vi "Log VNA Data - mat.vi"(4 "error in (no error)":errorcluster, 7 "Data in":T1 {"LogStartTime" format="%<%x %.3X>T"}) -> (0 "error out":errorcluster, 3 "Data out":T1 {"LogStartTime" format="%<%x %.3X>T"})   [LabVIEW 2023]
uses:
  controls/UI Data.ctl
  <vilib>/NI/Modbus Library/API/Master/Modbus Master.lvclass
  LibreVNA/LibreVNA.lvclass
  <vilib>/Platform/storage/Storage.llb/usiSequenceRepresentation.ctl
  <vilib>/Platform/storage/lvStorage.llb/_createOrGetByNameExplicitChildObject.vi
  <vilib>/Platform/storage/Storage.llb/__savePropString.vi
  <vilib>/Platform/storage/lvStorage.llb/xStorage/xStorageSupp/ErrorOut.vi
  <vilib>/Platform/storage/lvStorage.llb/_saveFloat64Channel.vi
  <vilib>/Platform/storage/lvStorage.llb/xStorage/Write Data/Write Data.xnode
panel:
  out "resulting string":string
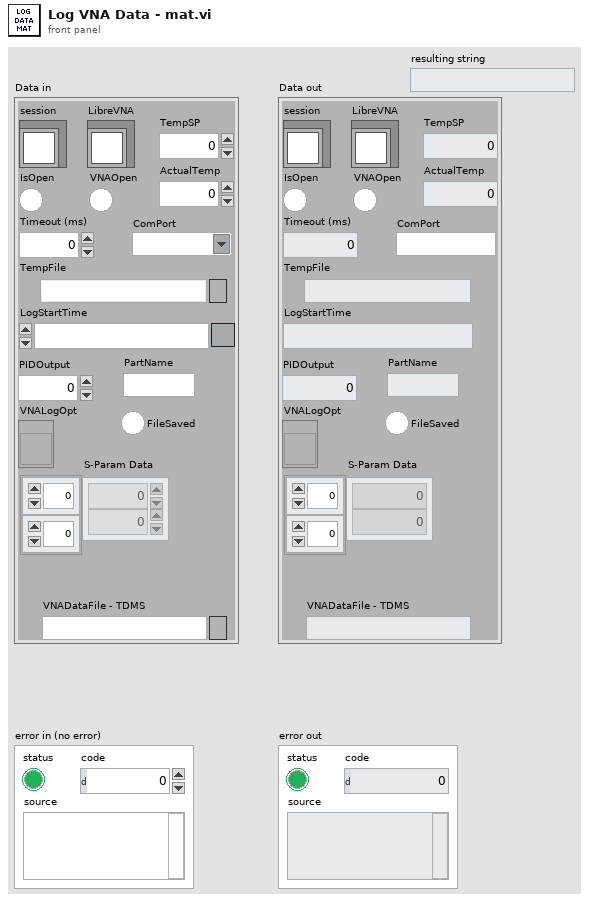
[diagram p1: front panel]
types:
  T1 = typedef "UI Data.ctl" = cluster{"session":refnum<class "Modbus Master.lvclass">, "IsOpen":bool, "Timeout (ms)":i32, "TempFile":path, "LogStartTime":timestamp, "LibreVNA":refnum<class "LibreVNA.lvclass">, "VNAOpen":bool, "TempSP":dbl, "ActualTemp":dbl, "FileSaved":bool, "PIDOutput":dbl, "VNALogOpt":refnum<vi>, "PartName":string, "ComPort":refnum<visa-resource-name>, "S-Param Data":dbl[][], "VNADataFile - TDMS":path}
  T2 = enum16{"Append values", "Replace values at index", "Replace all values"}
  T3 = enum16{"UPDATE", "READ", "QUERY", "CREATE CHILD", "CREATE", "CONNECT", "DISCONNECT"}
  T4 = typedef "usiSequenceRepresentation.ctl" = enum16{"explicit", "implicit"}
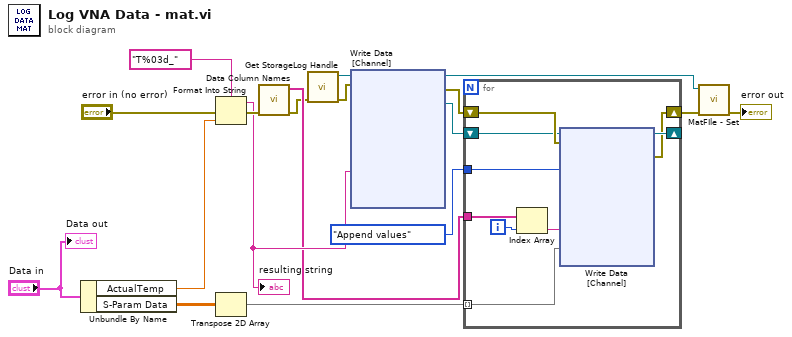
[diagram p0: block diagram]
diagram:
  n1 = Unbundle By Name("Data in") -> ("ActualTemp"=w17:dbl, "S-Param Data"=w15:dbl[][])
  n2 = Format Into String(format string="T%03d_", error in="error in (no error)", w17) -> (resulting string=w10:string, error out=w13:errorcluster)  [unwired: 1 in]
  "resulting string" <- w10
  n3 = Transpose 2D Array(2D array=w15) -> (transposed array=w9:dbl[][])
  n4 = call "Data Column Names.vi"("error in"=w13) -> ("error out"=w1:errorcluster, "Array"=w2:string[])  [unwired: 5 in]
  n5 = call "Get StorageLog Handle.vi"("error in"=w1) -> ("error out"=w11:errorcluster, "storage refnum (file) out"=w12:refnum<k20>)  [unwired: 4 in, 1 out]
  n6 = xnode "Write Data\n[Channel]"("Name"=w10, "storage refnum (file)"=w12, "error in"=w11) -> ("storage refnum (file) out"=w5:refnum<k20>, "error out"=w7:errorcluster, "storage refnum (channel group)"=w8:refnum<k20>)  [unwired: 1 in]
  n7 = for {
    tunnel: w9 -> [w19] mode=indexing
    shift-right: [w23] -> _
    shift-left: w8 -> [w24]
    tunnel: T2."Append values" ("append / replace (append data values)") -> [w21]
    shift-right: [w22] -> w4
    shift-left: w7 -> [w25]
    tunnel: w2 -> [w27]
    i -> [w26]
    n8 = Index Array(array=w27, index=w26) -> (element=w20:string)
    n9 = xnode "Write Data\n[Channel]"("Name"=w20, "Signal"=w19, "storage refnum (channel group)"=w24, "error in"=w25, "append / replace (append data values)"=w21) -> ("storage refnum (channel group) out"=w23:refnum<k20>, "error out"=w22:errorcluster)  [unwired: 1 in, 1 out]
  }
  n10 = call "MatFIle - Set.vi"("error in"=w4, "storage refnum (file) in"=w5) -> ("error out"=→"error out":errorcluster)  [unwired: 3 in, 2 out]
  "Data out" <- "Data in"
